vi "Update Waypoints.vi"(6 "Waypoints":T2, 9 "Tangents":cluster{sgl, sgl}[](array[cluster]), 10 "Drive Type":T1, 11 "X":dbl[](array[numeric])) -> (3 "Updated Waypoints":cluster{"x":dbl, "y":dbl, "th":dbl}[](array[cluster]))   [LabVIEW 2025]
uses:
  Bezier/Types/Waypoints.ctl
  Types/Drive Type.ctl
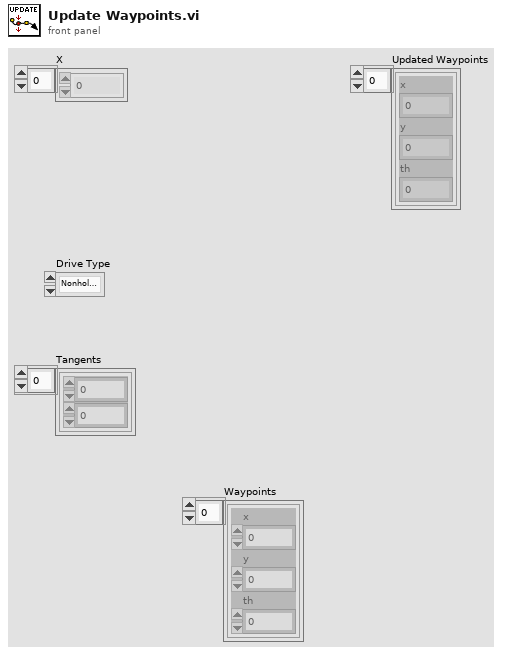
[diagram p1: front panel]
types:
  T1 = typedef "Drive Type.ctl" = enum16{"Nonholonomic", "Holonomic"}
  T2 = typedef "Waypoints.ctl" = cluster{"x":sgl, "y":sgl, "th":sgl}[]
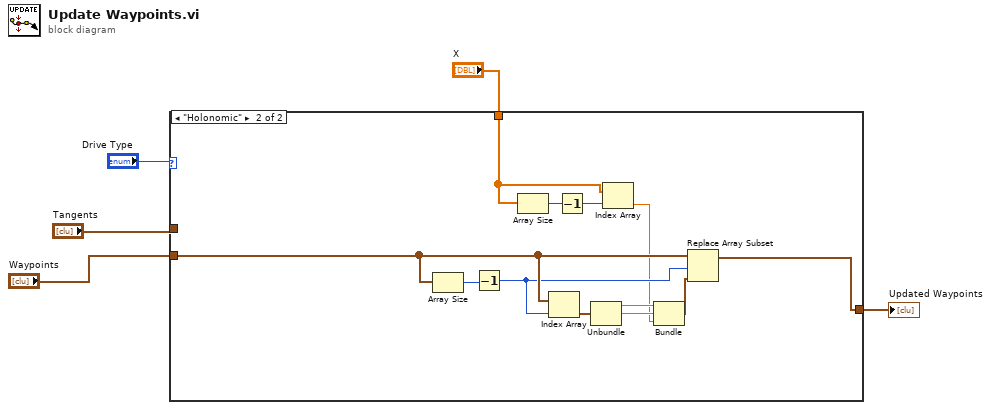
[diagram p0: block diagram]
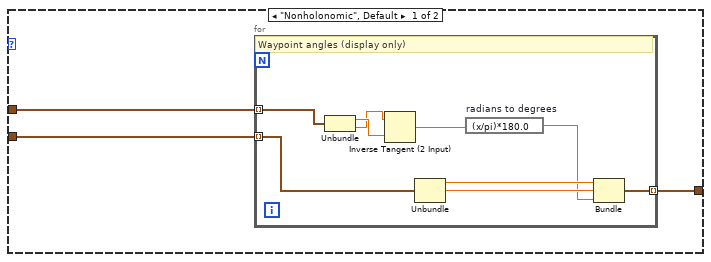
[diagram p2: hidden frame]
diagram:
  n1 = case shown="\"Holonomic\"" "Drive Type" {
    tunnel: "Tangents" -> [w8 _]
    tunnel: "Waypoints" -> [w7 w25]
    tunnel: [w6 w18] -> w3
    tunnel: "X" -> [_ w27]
    frame "Nonholonomic", Default {
      n2 = for {
        tunnel: w7 -> [w17] mode=indexing
        tunnel: w8 -> [w9] mode=indexing
        tunnel: [w14] -> w6 mode=indexing
        # "Waypoint angles (display only)"
        n3 = Unbundle(w9) -> (w12:sgl, w11:sgl)
        n4 = Inverse Tangent (2 Input)(1:w12, 2:w11) -> (0:w10:sgl)
        n5 = Unbundle(w17) -> ("x"=w16:sgl, "y"=w15:sgl)  [unwired: 1 out]
        n6 = expression code="(x/pi)*180.0" "radians to degrees"(w10) -> (w13:sgl)
        n7 = Bundle("x"=w16, "y"=w15, w13) -> (w14:cluster{"x":sgl, "y":sgl, sgl})  [unwired: 1 in]
      }
    }
    frame "Holonomic" {
      n8 = Array Size(array=w25) -> (size(s)=w26:i32)
      n9 = Decrement(x=w26) -> (x-1=w24:i32)
      n10 = Array Size(array=w27) -> (size(s)=w29:i32)
      n11 = Index Array(array=w25, index=w24) -> (element=w23:cluster{"x":sgl, "y":sgl, "th":sgl})
      n12 = Decrement(x=w29) -> (x-1=w28:i32)
      n13 = Unbundle(w23) -> ("x"=w22:sgl, "y"=w21:sgl)  [unwired: 1 out]
      n14 = Index Array(array=w27, index=w28) -> (element=w20:dbl)
      n15 = Bundle("x"=w22, "y"=w21, w20) -> (w19:cluster{"x":sgl, "y":sgl, dbl})  [unwired: 1 in]
      n16 = Replace Array Subset(array=w25, new element=w19, index=w24) -> (w18:T2)
    }
  }
  "Updated Waypoints" <- w3
